vi "Setup Window.vi"(8 "error in (no error)":errorcluster, 10 "Camera Controller":enum16{"None", "Spherical", "Flying"}(ring), 11 "Window State":T1(ring)) -> (0 "error out":errorcluster, 3 "New Window Refnum":refnum<vi>)   [LabVIEW 2020, in "NI_3D Picture Control.lvlib"]
doc: "Creates a new window with hardware acceleration for rendering the 3D scene."
uses:
  NI_3D Picture Control.lvlib
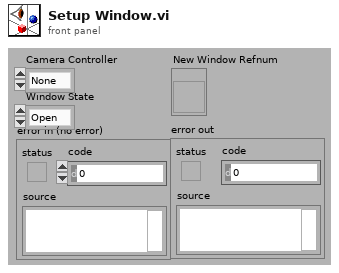
[diagram p1: front panel]
types:
  T1 = enum16{"Open", "Minimized", "Maximized", "Hidden"}
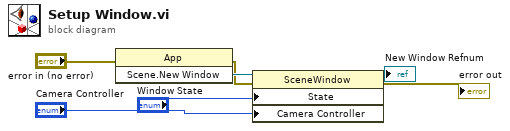
[diagram p0: block diagram]
diagram:
  n1 = invoke class="App" method="Scene.New Window"(error in="error in (no error)") -> (error out=w5:errorcluster, "Scene.New Window"=w6:refnum<vi>)  [unwired: 2 in, 1 out]
  n2 = property class="SceneWindow"(reference=w6, error in=w5, "State"="Window State", "Camera Controller"="Camera Controller") -> (reference out=→"New Window Refnum":refnum<vi>, error out=→"error out":errorcluster)
